vi "Alumina Material Properties.vi"(6 "m-nm Al2O3":dbl, 9 "Alumina Thickness":dbl, 10 "Energy (Heat; I^2R)":dbl, 11 "NS Base Area":dbl) -> (1 "Volume Al2O3":dbl, 2 "Delta Temp Change Al2O3":dbl, 3 "Mass Al2O3":dbl, 4 "Al2O3 Thickness":dbl, 5 "Al2O3 Specfic Heat Capacity":dbl, 7 "Al2O3 Density":dbl)   [LabVIEW 2020]
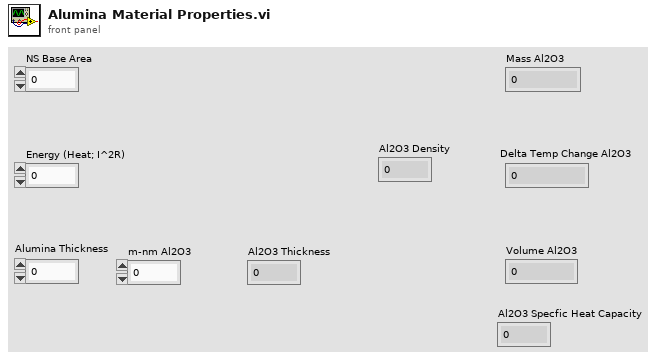
[diagram p1: front panel]
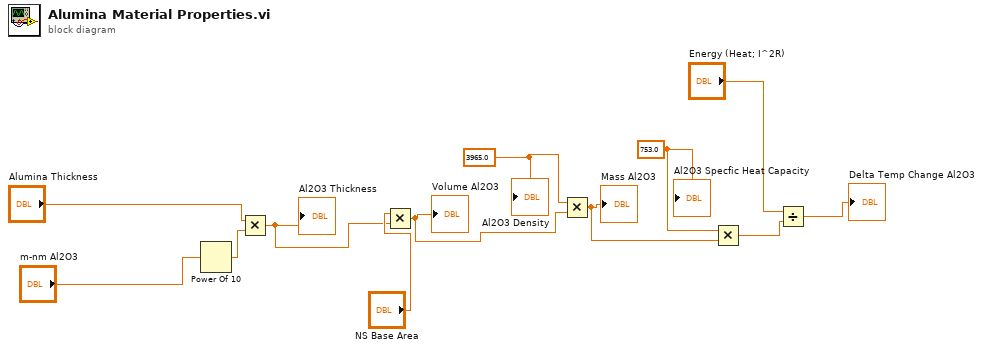
[diagram p0: block diagram]
diagram:
  w11 = 753.0 ("Silicon Specfic Heat Capacity 4")
  w6 = 3965.0 ("Silicon Density 4")
  n1 = Power Of 10(x="m-nm Al2O3") -> (10^x=w1:dbl)
  n2 = Multiply(x="Alumina Thickness", y=w1) -> (x*y=w4:dbl)
  "Al2O3 Thickness" <- w4
  n3 = Multiply(x="NS Base Area", y=w4) -> (x*y=w5:dbl)
  "Volume Al2O3" <- w5
  n4 = Multiply(x=w6, y=w5) -> (x*y=w10:dbl)
  "Mass Al2O3" <- w10
  n5 = Multiply(x=w11, y=w10) -> (x*y=w12:dbl)
  n6 = Divide(x="Energy (Heat; I^2R)", y=w12) -> (x/y=→"Delta Temp Change Al2O3":dbl)
  "Al2O3 Density" <- w6
  "Al2O3 Specfic Heat Capacity" <- w11
